vi "03.2 Analyze Threshold(SubVI).vi"(8 "Error In":errorcluster, 10 "Threshold (RMS)":dbl, 11 "Data":dbl[][](array[numeric])) -> (0 "Error Out":errorcluster, 2 "Threshold exceeded?":bool, 3 "RMS Results per Channel":dbl[](array[numeric]))   [LabVIEW 2019]
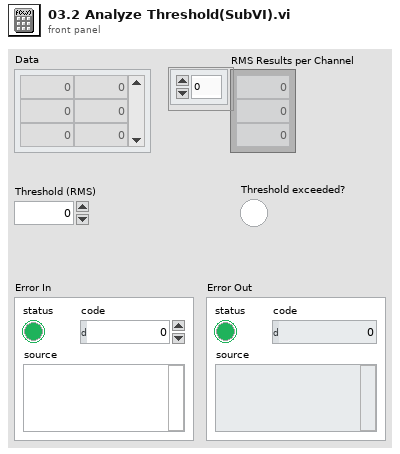
[diagram p1: front panel]
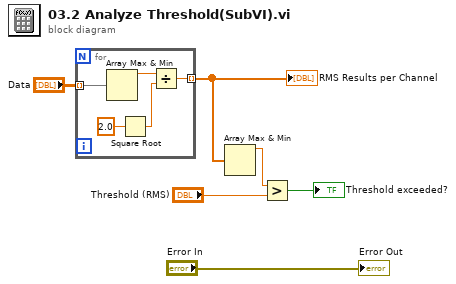
[diagram p0: block diagram]
diagram:
  n1 = for {
    tunnel: "Data" -> [w11] mode=indexing
    tunnel: [w7] -> w4 mode=indexing
    n2 = Array Max & Min(array=w11) -> (max value=w8:dbl)  [unwired: 3 out]
    n3 = Square Root(x=2.0) -> (sqrt(x)=w9:dbl)
    n4 = Divide(x=w8, y=w9) -> (x/y=w7:dbl)
  }
  "RMS Results per Channel" <- w4
  n5 = Array Max & Min(array=w4) -> (max value=w3:dbl)  [unwired: 3 out]
  n6 = Greater?(x=w3, y="Threshold (RMS)") -> (0:→"Threshold exceeded?":bool)
  "Error Out" <- "Error In"
